vi "Check if configuration files exist.vi"(8 "error in (no error)":errorcluster, 11 "Cascade512IIBase in":refnum<class "DAQCascade512II.lvclass">) -> (0 "error out":errorcluster, 2 "configuration file exists?":bool, 3 "Cascade512IIBase out":refnum<class "DAQCascade512II.lvclass">)   [LabVIEW 2012, in "DAQCascade512II.lvclass"]
doc: "Checks whether all required configuration files for the component tree exists."
uses:
  DAQCascade512II.lvclass
  <vilib>/Distrio/Murmex/Murmex/Murmex.lvclass
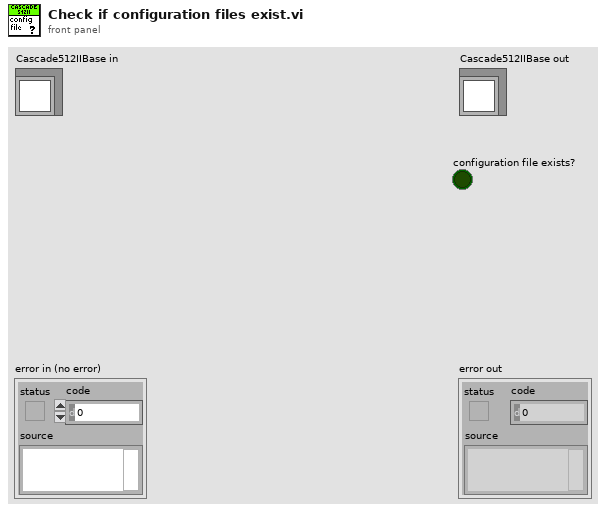
[diagram p1: front panel]
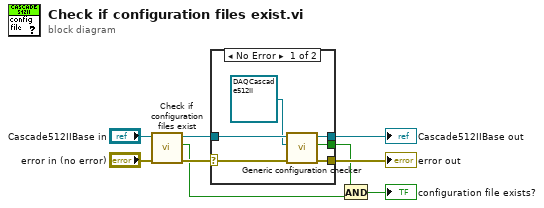
[diagram p0: block diagram]
diagram:
  n1 = call-parent "Check if configuration files exist.vi"("error in (no error)"="error in (no error)", "MurmexBase in"="Cascade512IIBase in") -> ("error out"=w7:errorcluster, "configuration file exists?"=w3:bool, "MurmexBase out"=w6:refnum<class "DAQCascade512II.lvclass">)  [unwired: 7 in]
  n2 = case shown="No Error" w7 {
    selector: w7 -> [w15 w17]
    tunnel: [w14 w17] -> w4
    tunnel: w6 -> [w13 w16]
    tunnel: [w12 w16] -> w5
    tunnel: [w11 _] -> w1
    frame No Error {
      n3 = call <vilib>:"Generic configuration checker.vi"("error in (no error)"=w15, "inheritance level"=refnum<class "DAQCascade512II.lvclass"> refnum ("DAQCascade512II"), "Murmex in"=w13) -> ("error out"=w14:errorcluster, "configuration file exists?"=w11:bool, "Murmex out"=w12:refnum<class "DAQCascade512II.lvclass">)  [unwired: 6 in]
    }
    frame Error {
    }
  }
  "error out" <- w4
  "Cascade512IIBase out" <- w5
  n4 = And(x=w1, y=w3) -> (x .and. y?=→"configuration file exists?":bool)
